vi "RT_RW_2ADC_W_DACs_FPGA_CLKthenWrite.vi"() -> ()   [LabVIEW 2018]
uses:
  <vilib>/FPGAPlugInAG/myRIO-1900/niLvFpga_Open_myRIO-1900.vi
  <vilib>/rvi/interface/common/dynamic/niFpgaDynamicAddResources.vi
  <vilib>/Utility/error.llb/Error Cluster From Error Code.vi
  <vilib>/rvi/errors/niLvFpgaAdjustHostInterfaceError.vi
  <vilib>/FPGAPlugInAG/Dynamic/niLvFpga_Close_Dynamic.vi
  <vilib>/rvi/interface/nirviOpenFPGA/nirviOpenFPGA.xnode
  FPGA Bitfiles/ASPE2019amplifie_FPGATarget_fpgaW&RADCsW3DAC_cQtLOI3gdQI.lvbitx
  FPGA files/fpga_W&R_ADCs_W_3DAC_CLK_then_Write.vi
  <vilib>/rvi/interface/nirviReadWriteControl/nirviReadWriteControl.xnode
  <vilib>/rvi/interface/nirviCloseFPGA/nirviCloseFPGA.xnode
  NiFpgaLv.dll
  <vilib>/rvi/interface/Simulation/niFpgaSimulationCallBeginRW.vi
panel:
  in  "milliseconds to wait":u32
  out "CH1 (V) 2":dbl(graph)=-0.3778018523887268
  in  "ADC 1 write":bool[](array[boolean])=[FALSE, FALSE, FALSE, FALSE, FALSE, TRUE, FALSE, FALSE, FALSE, FALSE, FALSE, FALSE, FALSE, FALSE, FALSE, FALSE]
  in  "ADC 2 write":bool[](array[boolean])=[FALSE, FALSE, FALSE, FALSE, FALSE, TRUE, FALSE, FALSE, FALSE, FALSE, FALSE, FALSE, FALSE, FALSE, FALSE, FALSE]
  out "loop rate (kHz)":dbl
  in  "DAC (V)":dbl
  in  "Stop Button":bool
  out "CH1 (V)":u16(graph)
  # "Both channels are configured to read +/-10 V range in differential mode"
  # "If I change the below bits to CH2, signal looks noisy"
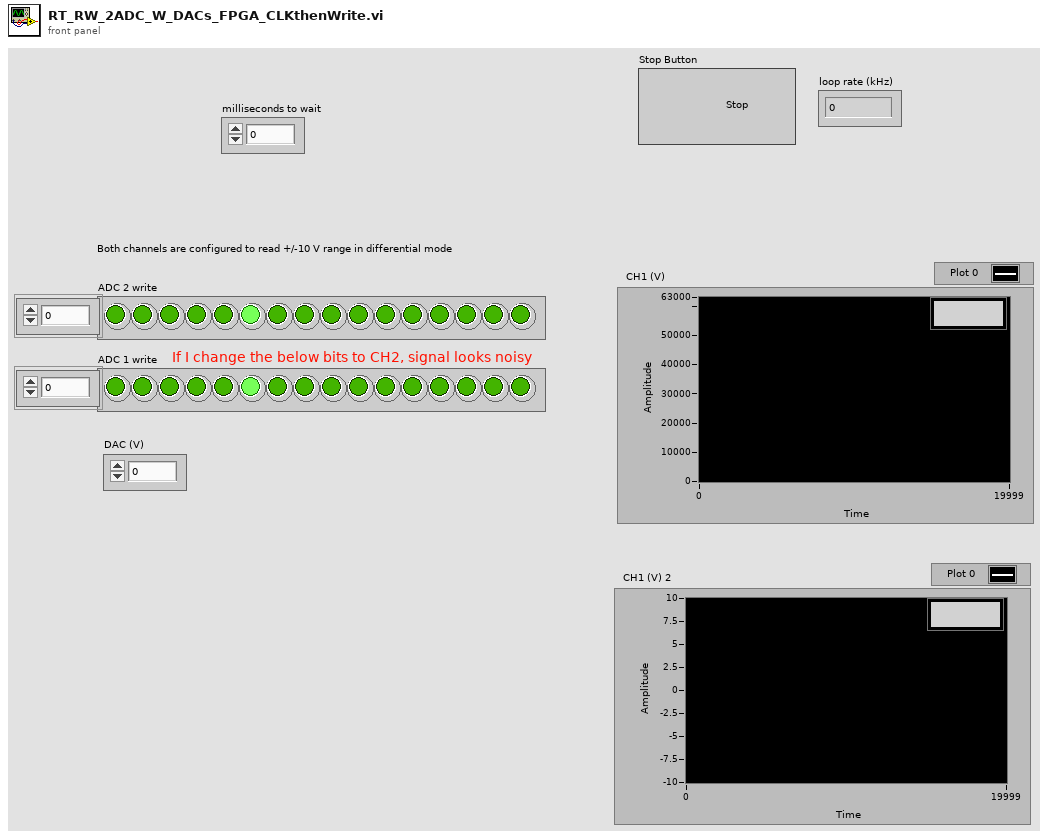
[diagram p1: front panel]
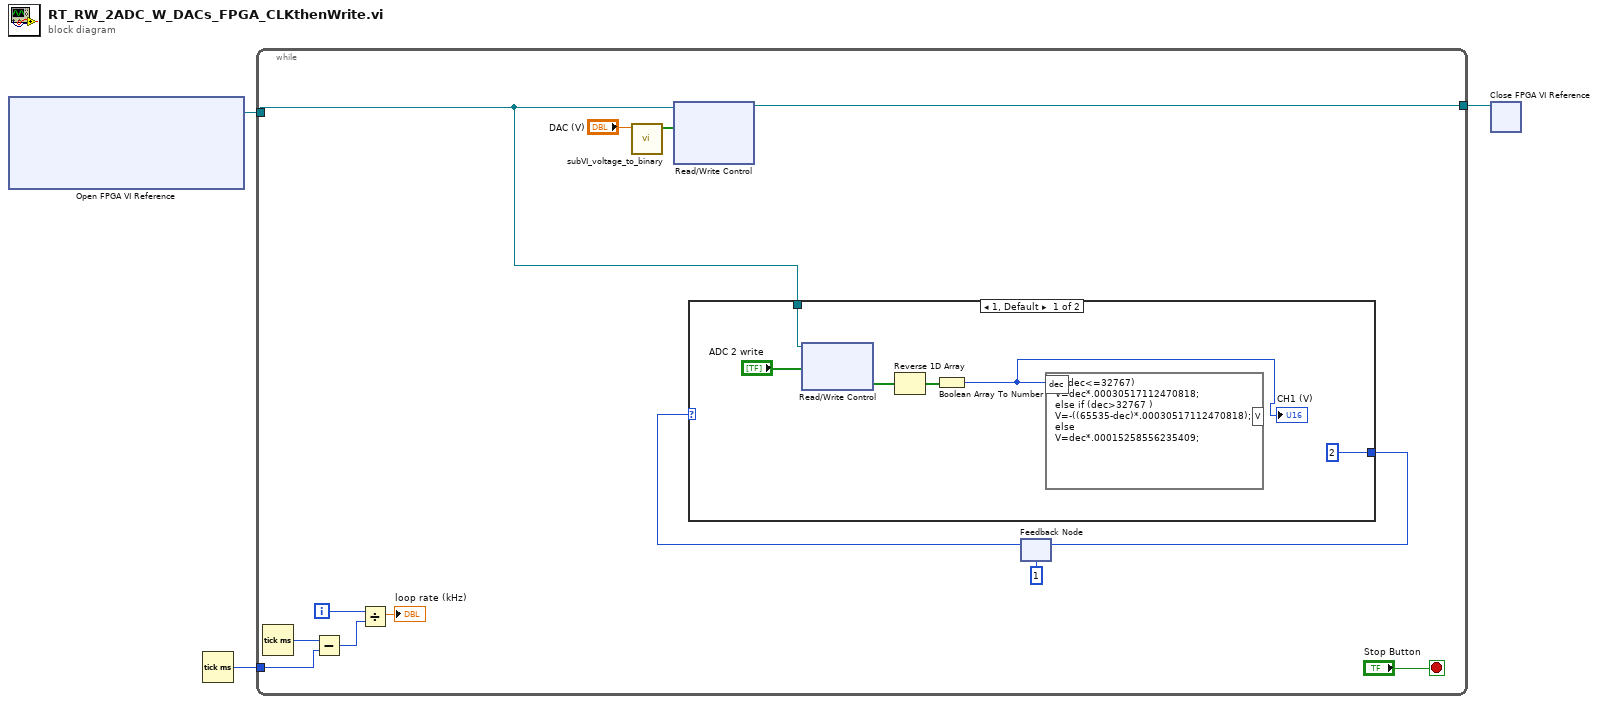
[diagram p0: block diagram]
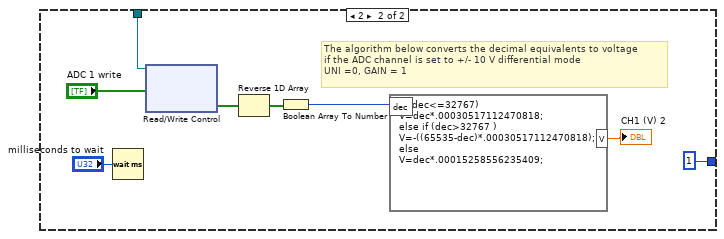
[diagram p2: hidden frame]
diagram:
  n1 = xnode "Open FPGA VI Reference"() -> ("FPGA VI Reference Out"=w3:refnum<k20>)  [unwired: 2 in, 1 out]
  n2 = Tick Count (ms)() -> (millisecond timer value=w2:u32)
  n3 = while {
    tunnel: w3 -> [w4]
    tunnel: w2 -> [w14]
    tunnel: [w5] -> w1
    i -> [w13]
    stop <- "Stop Button" stop-if-true
    n4 = Tick Count (ms)() -> (millisecond timer value=w15:u32)
    n5 = Subtract(x=w15, y=w14) -> (x-y=w12:u32)
    n6 = Divide(x=w13, y=w12) -> (x/y=→"loop rate (kHz)":dbl)
    n7 = call "subVI_voltage_to_binary.vi"("voltage"="DAC (V)") -> ("binary"=w7:bool[])  [unwired: 10 in]
    n8 = xnode "Read/Write Control"("FPGA VI Reference In"=w4, "DAC 1 write"=w7) -> ("FPGA VI Reference Out"=w5:refnum<k20>)  [unwired: 3 in, 1 out]
    n9 = feedback #1(u8 1) -> (w9:u8)
    n10 = case shown="1, Default" w9 {
      tunnel: [u8 2 u8 1] -> w6
      tunnel: w4 -> [w18 w24]
      frame 1, Default {
        n11 = xnode "Read/Write Control"("FPGA VI Reference In"=w18, "ADC write"="ADC 2 write") -> ("ADC read"=w21:bool[])  [unwired: 1 in, 2 out]
        n12 = Reverse 1D Array(array=w21) -> (reversed array=w19:bool[])
        n13 = Boolean Array To Number(Boolean array=w19) -> (number=w17:u16)
        "CH1 (V)" <- w17
        n14 = formula code="if (dec<=32767)\nV=dec*.00030517112470818;\nelse if (dec>32767 )\nV=-((65535-dec)*.00030517112470818);\nelse\nV=dec*.00015258556235409;"("dec"=w17) -> ()  [unwired: 1 out]
      }
      frame 2 {
        # "The algorithm below converts the decimal equivalents to voltage\nif the ADC channel is set to +/- 10 V differential mode\nUNI =0, GAIN = 1"
        n15 = Wait (ms)(milliseconds to wait="milliseconds to wait") -> ()  [unwired: 1 out]
        n16 = xnode "Read/Write Control"("FPGA VI Reference In"=w24, "ADC write"="ADC 1 write") -> ("ADC read"=w28:bool[])  [unwired: 1 in, 2 out]
        n17 = Reverse 1D Array(array=w28) -> (reversed array=w26:bool[])
        n18 = Boolean Array To Number(Boolean array=w26) -> (number=w30:u16)
        n19 = formula code="if (dec<=32767)\nV=dec*.00030517112470818;\nelse if (dec>32767 )\nV=-((65535-dec)*.00030517112470818);\nelse\nV=dec*.00015258556235409;"("dec"=w30) -> ("V"=→"CH1 (V) 2":dbl)
      }
    }
    n20 = feedback-in #1(w6) -> ()
  }
  n21 = xnode "Close FPGA VI Reference"("FPGA VI Reference In"=w1) -> ()  [unwired: 1 in, 1 out]
